vi "ConnectandDisconnect.vi"(0 "error in":errorcluster {"code" format="%.0x"}, 1 "Virtual Device Name":string="SwitchConfiguration1", 2 "Option String (\"\")":string, 3 "Connection Specification (\"\")":string, 4 "Disconnection Specification (\"\")":string) -> (20 "Status":string, 27 "error out":errorcluster {"code" format="%.0x"})   [LabVIEW 2021, in "SimpleSwitch_Reusables.lvlib"]
uses:
  SimpleSwitch_Reusables.lvlib
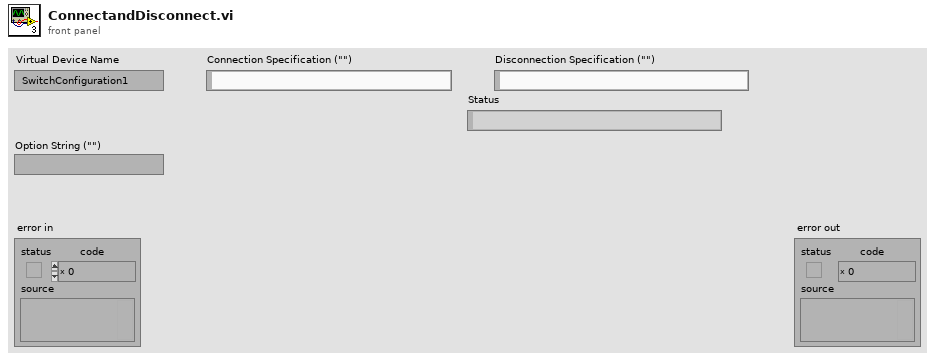
[diagram p1: front panel]
types:
  T1 = typedef "niSE SessionRefnum.ctl" = refnum<k1>
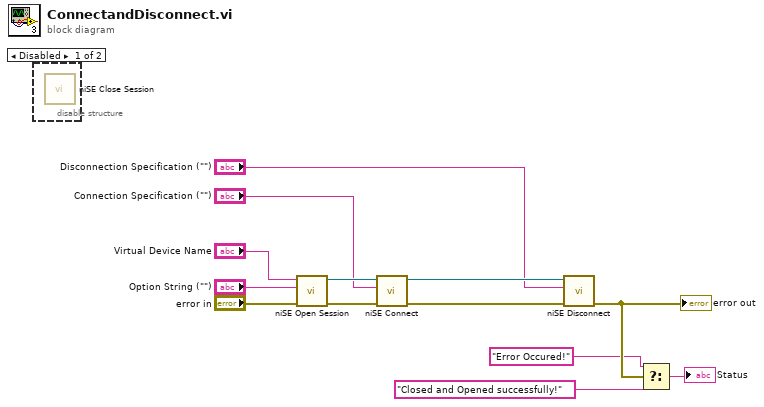
[diagram p0: block diagram]
diagram:
  n1 = disable-structure shown="Disabled" {
    frame Disabled {
      n2 = call <vilib>:"niSE Close Session.vi"() -> ()  [unwired: 7 in, 1 out]
    }
    frame Enabled {
    }
  }
  n3 = call <vilib>:"niSE Open Session.vi"("error in (no error)"="error in", "Option String (\"\")"="Option String (\"\")", "Virtual Device Name (SwitchConfiguration1)"="Virtual Device Name") -> ("error out"=w11:errorcluster, "NISE Session (out)"=w13:T1)  [unwired: 3 in]
  n4 = call <vilib>:"niSE Connect.vi"("error in (no error)"=w11, "Connection Specification (\"\")"="Connection Specification (\"\")", "NISE Session (in)"=w13) -> ("error out"=w10:errorcluster, "NISE Session (out)"=w12:T1)  [unwired: 7 in]
  n5 = call <vilib>:"niSE Disconnect.vi"("error in (no error)"=w10, "Disconnection Specification (\"\")"="Disconnection Specification (\"\")", "NISE Session (in)"=w12) -> ("error out"=w3:errorcluster)  [unwired: 3 in, 1 out]
  "error out" <- w3
  n6 = Select(t="Error Occured!" ("Connection Specification (\"\")"), s=w3, f="Closed and Opened successfully!" ("Connection Specification (\"\")")) -> (s? t:f=→"Status":string)
